vi "GetAvailableDemoCameraModels.vi"(8 "error in (no error)":errorcluster) -> (0 "error out":errorcluster, 1 "model_count":i32, 2 "model_array":i32[](array[numeric]))   [LabVIEW 2019, in "PICam.lvlib"]
uses:
  PICam.lvlib
  Ctrls/PicamErrors.ctl
  Picam64.dll
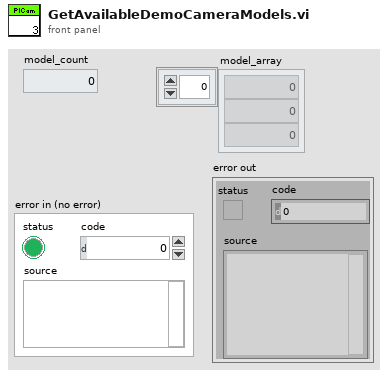
[diagram p1: front panel]
types:
  T1 = typedef "PICam.lvlib/PicamErrors.ctl" = i32
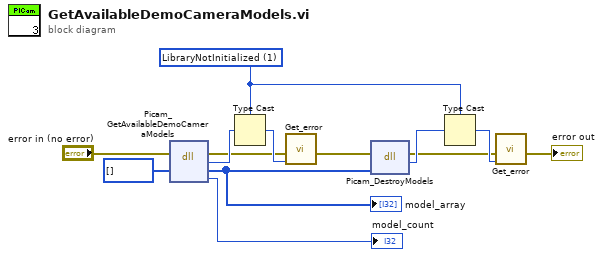
[diagram p0: block diagram]
diagram:
  w3 = T1 1 items=["LibraryNotInitialized"=1, "InvalidParameterValue"=2, "UnexpectedNullPointer"=3, "UnexpectedError"=4, "LibraryAlreadyInitialized"=5, "InvalidDemoModel"=6, "CameraAlreadyOpened"=7, "InvalidCameraID"=8, "InvalidHandle"=9, "ParameterValueIsReadOnly"=10, "ParameterHasInvalidValueType"=11, "ParameterDoesNotExist"=12, "ParameterHasInvalidConstraintType"=13, "ParameterValueIsIrrelevant"=14, "DeviceCommunicationFailed"=15, "InvalidEnumeratedType"=16, "EnumerationValueNotDefined"=17, "NotDiscoveringCameras"=18, "AlreadyDiscoveringCameras"=19, "AcquisitionInProgress"=20, "InvalidDemoSerialNumber"=21, "DemoAlreadyConnected"=22, "DeviceDisconnected"=23, "DeviceOpenElsewhere"=24, "ParameterIsNotOnlineable"=25, "ParameterIsNotReadable"=26, "AcquisitionNotInProgress"=27, "InvalidParameterValues"=28, "ParametersNotCommitted"=29, "InvalidAcquisitionBuffer"=30, "InsufficientMemory"=31, "TimeOutOccurred"=32, "AcquisitionUpdatedHandlerRegistered"=33, "NoCamerasAvailable"=34, "InvalidPointer"=35, "InvalidReadoutCount"=36, "InvalidReadoutTimeOut"=37, "InvalidConstraintCategory"=38, "InvalidCount"=39, "DemoNotSupported"=40, "NondestructiveReadoutEnabled"=41, "InvalidOperation"=42, "OperationCanceled"=43, "InvalidAcquisitionState"=44, "NoAccessoriesAvailable"=45, "AccessoryAlreadyOpened"=46, "InvalidAccessoryID"=47, "NotDiscoveringAccessories"=48, "AlreadyDiscoveringAccessories"=49, "ParameterIsNotWaitableStatus"=50, "InvalidWaitableStatusParameterTimeOut"=51, "ShutterOverheated"=52, "CameraFaulted"=53, "CenterWavelengthFaulted"=54] ("PICam_Error")
  n1 = dll-call lib="Picam*.*" fn="Picam_GetAvailableDemoCameraModels"(error in="error in (no error)", "model_array"=i32[] []) -> (error out=w9:errorcluster, "error"=w12:i32, "model_array"=w7:i32[], "model_count"=→"model_count":i32)  [unwired: 3 in, 1 out]
  "model_array" <- w7
  n2 = Type Cast(type=w3, x=w12) -> (*(type *) &x=w13:T1)
  n3 = call "Get_error.vi"("PICam_Error"=w13, "error in (no error)"=w9) -> ("error out"=w8:errorcluster)  [unwired: 9 in]
  n4 = dll-call lib="Picam*.*" fn="Picam_DestroyModels"(error in=w8, "model_array"=w7) -> (error out=w2:errorcluster, "error"=w6:i32)  [unwired: 3 in, 1 out]
  n5 = Type Cast(type=w3, x=w6) -> (*(type *) &x=w5:T1)
  n6 = call "Get_error.vi"("PICam_Error"=w5, "error in (no error)"=w2) -> ("error out"=→"error out":errorcluster)  [unwired: 9 in]
